vi "Initialize.vi"(8 "error in (no error)":errorcluster, 9 "Msg Ref":refnum<vi>, 10 "Name":string, 11 "Filter Wheel Simulator in":refnum<class "Filter Wheel Simulator.lvclass">) -> (0 "error out":errorcluster, 3 "Filter Wheel Simulator out":refnum<class "Filter Wheel Simulator.lvclass">)   [LabVIEW 2024, in "Filter Wheel Simulator.lvclass"]
uses:
  Filter Wheel Simulator.lvclass
  Filter Wheel cluster Simulated Status.ctl
  Filter Wheel Simulator.lvclass/Filter Wheel Simulator.ctl
  Filter Wheel Object/Filter Wheel.lvclass
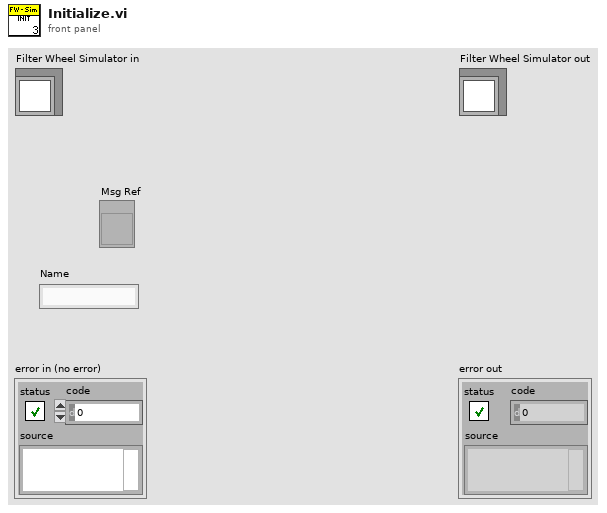
[diagram p1: front panel]
types:
  T1 = typedef "Filter Wheel Simulator.lvclass/Filter Wheel cluster Simulated Status.ctl" = cluster{"Move Start Time":timestamp, "Moving?":bool, "Target Pos":dbl, "Direction":bool}
  T2 = typedef "Filter Wheel.lvclass/Filter Wheel configuration.ctl" = cluster{"Num Wheels":i32, "Filters":T3[], "Invalid Combinations":i32[][], "Addr":refnum<visa-resource-name>, "Name":string, "Simulate":bool, "Default Speed":u16, "Homing":T4[]}
  T3 = typedef "Filter Wheel.lvclass/Filter Wheel Details.ctl" = cluster{"Names":string[], "Relative Position":i32[], "Wheel Name":string, "Size":i32}
  T4 = typedef "Filter Wheel Arduino Homing cluster.ctl" = cluster{"Direction":bool, "Speed":i32, "Accel":i32, "Error Cnts":i32, "Homing Delta":i32}
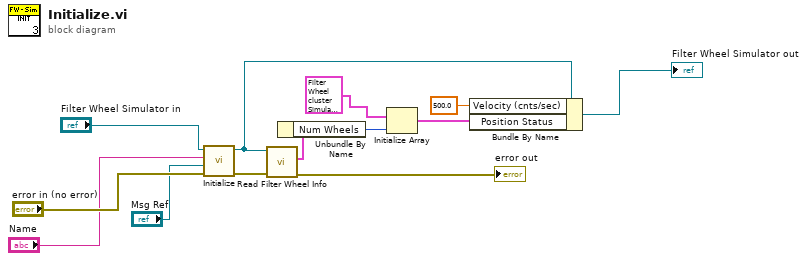
[diagram p0: block diagram]
diagram:
  n1 = call-parent "Initialize.vi"("error in (no error)"="error in (no error)", "Msg Ref"="Msg Ref", "Name"="Name", "Filter Wheel in"="Filter Wheel Simulator in") -> ("error out"=w8:errorcluster, "Filter Wheel out"=w9:refnum<class "Filter Wheel Simulator.lvclass">)  [unwired: 6 in]
  n2 = call-dynamic "Read Filter Wheel Info.vi"("error in (no error)"=w8, "Filter Wheel in"=w9) -> ("error out"=→"error out":errorcluster, "Filter Wheel Info"=w7:T2)  [unwired: 7 in, 1 out]
  n3 = Unbundle By Name(w7) -> ("Num Wheels"=w6:i32)
  n4 = Initialize Array(T1 {"Move Start Time"=timestamp(0 s since 1904-01-01), "Moving?"=FALSE, "Target Pos"=0.0, "Direction"=FALSE} ("Position Status"), w6) -> (w4:T1[])
  n5 = Bundle By Name(cluster=w9, "Velocity (cnts/sec)"=500.0, "Position Status"=w4) -> (→"Filter Wheel Simulator out":refnum<class "Filter Wheel Simulator.lvclass">)
